vi "Unit Test.vi"() -> ()   [LabVIEW 2018]
uses:
  PPLs/REST Interface/Parent/REST Interface.lvlibp/REST Interface.lvclass
  EnVision REST.lvclass
  C:/Projects/LabVIEW/PPLs/REST Interface/Parent/REST Interface.lvlibp/REST Interface.lvclass
  PPLs/REST Interface/Parent/REST Interface.lvlibp/Custom Controls/Request.ctl
  PPLs/REST Interface/Parent/REST Interface.lvlibp/Custom Controls/Headers.ctl
panel:
  in  "Single Header Name":string
  in  "Header":T1
  in  "Request":T2
  in  "Path (after URL)":string="service"
  out "error out":errorcluster
  out "Response":string
  out "Status Code":u16
  in  "error in (no error)":errorcluster
  in  "Base URL":string
  # "Unit Test"
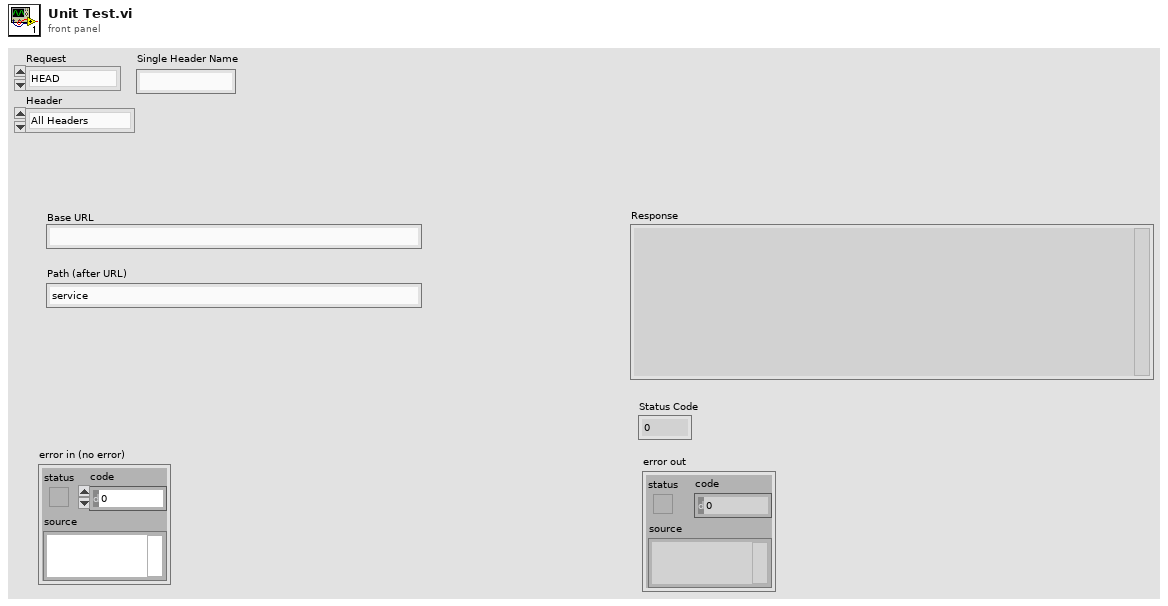
[diagram p1: front panel]
types:
  T1 = typedef "REST Interface.lvlibp/REST Interface.lvclass/Headers.ctl" = enum16{"All Headers", "Single Header"}
  T2 = typedef "REST Interface.lvlibp/REST Interface.lvclass/Request.ctl" = enum16{"HEAD", "PUT", "GET", "POST", "DELETE"}
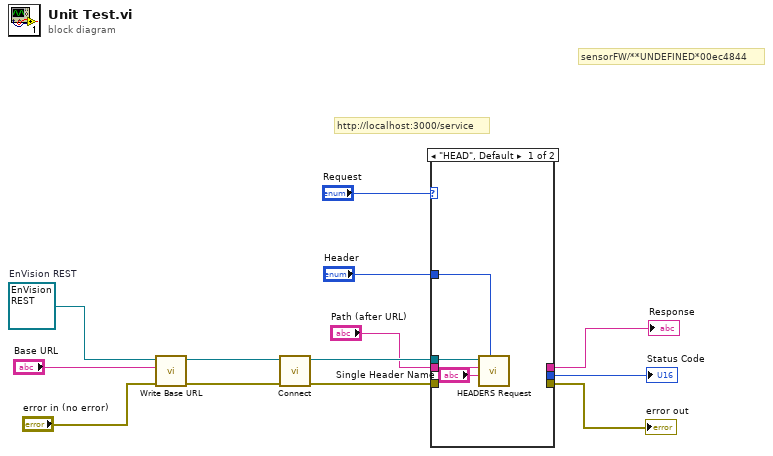
[diagram p0: block diagram]
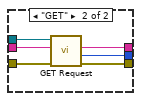
[diagram p2: hidden frame]
diagram:
  w3 = refnum<class "EnVision REST.lvclass"> refnum  # EnVision REST
  # "sensorFW/**UNDEFINED*00ec4844"
  # "http://localhost:3000/service"
  n1 = call "Write Base URL.vi"("error in (no error)"="error in (no error)", "Base URL"="Base URL", "REST Interface in"=w3) -> ("error out"=w10:errorcluster, "REST Interface out"=w11:refnum<class "EnVision REST.lvclass">)  [unwired: 7 in]
  n2 = call-dynamic "Connect.vi"("error in (no error)"=w10, "REST Interface in"=w11) -> ("error out"=w7:errorcluster, "REST Interface out"=w9:refnum<class "EnVision REST.lvclass">)  [unwired: 8 in]
  n3 = case shown="\"HEAD\", Default" "Request" {
    tunnel: w9 -> [w17 w23]
    tunnel: "Path (after URL)" -> [w16 w22]
    tunnel: w7 -> [_ w21]
    tunnel: [_ w20] -> w6
    tunnel: [_ w19] -> w5
    tunnel: [_ w18] -> w4
    tunnel: "Header" -> [w15 _]
    frame "HEAD", Default {
      n4 = call-dynamic "HEADERS Request.vi"("Header"=w15, "Single Header Name"="Single Header Name", "Path (after URL)"=w16, "EnVision REST in"=w17) -> ()  [unwired: 3 in, 5 out]
    }
    frame "GET" {
      n5 = call-dynamic "GET Request.vi"("error in (no error)"=w21, "Path (after URL)"=w22, "EnVision REST in"=w23) -> ("error out"=w18:errorcluster, "Status Code"=w20:u16, "Response"=w19:string)  [unwired: 5 in, 1 out]
    }
  }
  "Status Code" <- w6
  "Response" <- w5
  "error out" <- w4
